vi "npointrunavg.vi"(1 "n":i8, 2 "Input":dbl) -> (0 "Output":dbl)   [LabVIEW 2013]
uses:
  <vilib>/Analysis/baseanly.llb/Mean (DBL).vi
  <vilib>/Analysis/NI_AALBase.lvlib
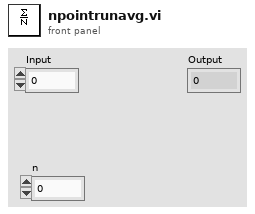
[diagram p1: front panel]
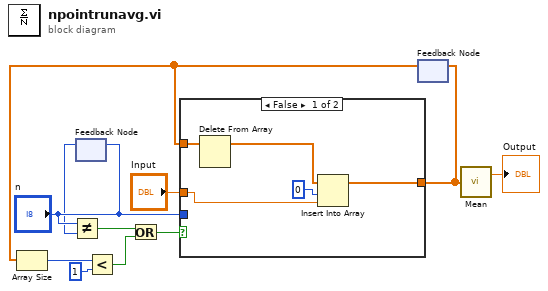
[diagram p0: block diagram]
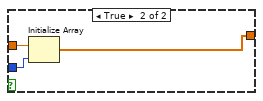
[diagram p2: hidden frame]
diagram:
  n1 = feedback #1() -> (w1:i8)  [unwired: 1 in]
  n2 = Not Equal?(x="n", y=w1) -> (x != y?=w6:bool)
  n3 = feedback-in #1("n") -> ()
  n4 = feedback #2() -> (w3:dbl[])  [unwired: 1 in]
  n5 = Array Size(array=w3) -> (size(s)=w10:i32)
  n6 = Less?(x=w10, y=1) -> (x < y?=w5:bool)
  n7 = Or(x=w6, y=w5) -> (x .or. y?=w7:bool)
  n8 = case shown="False" w7 {
    tunnel: "n" -> [_ w19]
    tunnel: "Input" -> [w14 w18]
    tunnel: [w13 w17] -> w4
    tunnel: w3 -> [w16 _]
    frame False {
      n9 = Delete From Array "Delete From Array"(array=w16) -> (array with subset deleted=w15:dbl[])  [unwired: 2 in, 1 out]
      n10 = Insert Into Array "Insert Into Array"(array=w15, index=0, new element=w14) -> (w13:dbl[])
    }
    frame True {
      n11 = Initialize Array "Initialize Array"(w18, w19) -> (w17:dbl[])
    }
  }
  n12 = feedback-in #2(w4) -> ()
  n13 = call-poly <vilib>:"Mean.vi"("X"=w4) -> ("mean"=→"Output":dbl)  [unwired: 1 out]
